vi "Get Device USB Strings.vi"(8 "error in (no error)":errorcluster, 10 "Device Index":u32, 11 "RTL-SDR in":refnum<class "RTL-SDR.lvclass">) -> (0 "error out":errorcluster, 1 "function return":i32, 2 "Device USB Strings":T1, 3 "RTL-SDR out":refnum<class "RTL-SDR.lvclass">)   [LabVIEW 2015, in "RTL-SDR.lvclass"]
doc: "Created IvanLis by LabVIEW Portal\nProfile: http://labviewportal.org/memberlist.php?mode=viewprofile&u=987\neMail: IvanLisanov@gMail.com\nTelegram: https://t.me/IvanLis"
uses:
  RTL-SDR.lvclass
  TypeDef/Device USB String.ctl
  RTL-SDR.lvclass/RTL-SDR.ctl
panel:
  in  "manufact":string
  in  "product":string
  in  "serial":string
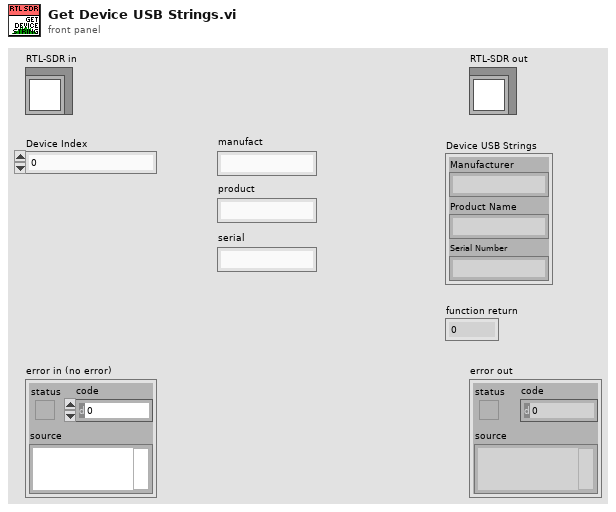
[diagram p1: front panel]
types:
  T1 = typedef "RTL-SDR.lvclass/Device USB String.ctl" = cluster{"Manufacturer":string, "Product Name":string, "Serial Number":string}
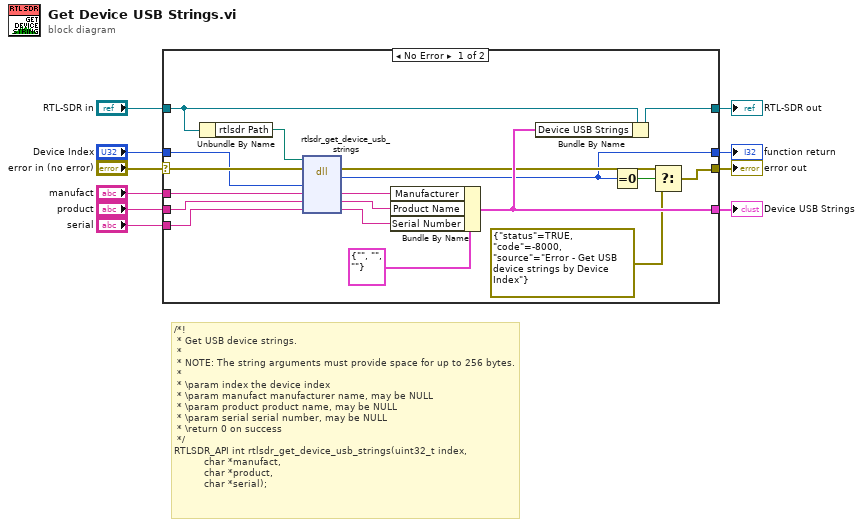
[diagram p0: block diagram]
diagram:
  # "/*!\n * Get USB device strings.\n *\n * NOTE: The string arguments must provide space for up to 256 bytes.\n *\n * \\param index the device index\n * \\param manufact manufacturer name, may be NULL\n * \\param product product name, may be NULL\n * \\param serial serial number, may be NULL\n * \\return 0 on success\n */\nRTLSDR_API int rtlsdr_get_device_usb_strings(uint32_t index,\n\t\t\t\t\t     char *manufact,\n\t\t\t\t\t     char *product,\n\t\t\t\t\t     char *serial);"
  n1 = case shown="No Error" "error in (no error)" {
    selector: "error in (no error)" -> [w28 w30]
    tunnel: [w13 w30] -> w9
    tunnel: [w17 w29] -> w7
    tunnel: "RTL-SDR in" -> [w26 w29]
    tunnel: "Device Index" -> [w27 _]
    tunnel: [w11 _] -> w5
    tunnel: "manufact" -> [w24 _]
    tunnel: "product" -> [w23 _]
    tunnel: "serial" -> [w22 _]
    tunnel: [w16 _] -> w1
    frame No Error {
      n2 = Unbundle By Name(w26) -> ("rtlsdr Path"=w25:path)
      n3 = dll-call lib="C:/Users/Ivan/Desktop/D-23-09-24 (RTL-SDR)/Project (Pelleng-SDR)/rtlsdr/dll/rtlsdr.*" fn="rtlsdr_get_device_usb_strings"(path in=w25, error in=w28, "index"=w27, "manufact"=w24, "product"=w23, "serial"=w22) -> (error out=w14:errorcluster, "return type"=w11:i32, "manufact"=w20:string, "product"=w19:string, "serial"=w18:string)  [unwired: 2 in, 1 out]
      n4 = Bundle By Name(cluster=T1 {"Manufacturer"="", "Product Name"="", "Serial Number"=""} ("Device USB Strings"), "Manufacturer"=w20, "Product Name"=w19, "Serial Number"=w18) -> (w16:T1)
      n5 = Bundle By Name(cluster=w26, "Device USB Strings"=w16) -> (w17:refnum<class "RTL-SDR.lvclass">)
      n6 = Equal To 0?(x=w11) -> (x = 0?=w12:bool)
      n7 = Select(t=w14, s=w12, f=errorcluster {"status"=TRUE, "code"=-8000, "source"="Error - Get USB device strings by Device Index"} ("error out")) -> (s? t:f=w13:errorcluster)
    }
    frame Error {
    }
  }
  "error out" <- w9
  "RTL-SDR out" <- w7
  "function return" <- w5
  "Device USB Strings" <- w1
